vi "FPGA Main_SPI API with Waveform Library.vi"() -> ()   [LabVIEW 2014]
uses:
  <userlib>/_NI SPI IP/FPGA/Controllers/Public/Transfer Settings.ctl
  <vilib>/Platform/TimedLoop/XDataNode/timing_clust.ctl
  <vilib>/Platform/TimedLoop/XDataNode/nitl_modes.ctl
  <vilib>/Platform/TimedLoop/XDataNode/wakeup.ctl
  <vilib>/SPI API/SPIAPI/DIO/SPI Digital IO Lines.ctl
  <vilib>/SPI API/SPIAPI/DIO/SPI DIO Enable Lines.ctl
  <vilib>/rvi/Emulation/niFpgaGetClockAttributes.vi
  <vilib>/rvi/Emulation/niFpgaSctlEmulationGetInTimedLoop.vi
  <vilib>/rvi/Emulation/niFpgaEmulationReportErrorSimple.vi
  <vilib>/rvi/Emulation/niFpgaProcessEmulError.vi
  <vilib>/rvi/Emulation/niFpgaCriticalErrorInLSC.vi
  <vilib>/rvi/interface/RandomDataEmulation/niFpgaRandomDataHandleErrors.vi
  <vilib>/Platform/TimedLoop/XDataNode/XDataNode.xnode
  <vilib>/rvi/DataTransferAndStorage/Container/XNode/niFpgaContainer.xnode
  <vilib>/rvi/interface/RandomDataEmulation/nirviRandomDataFpgaReadWriteTemplate.vi
  <vilib>/Platform/TimedLoop/XDataNode/XDNodeRunTimeDep.lvlib
  <userlib>/_NI SPI IP/FPGA/Controllers/NI SPI IP FPGA.lvlib
panel:
  in  "SPI PHY Settings":T1={"Divide Value"=10, "Transfer Length (bits)"=16, "CS Asserted Polarity"=FALSE, "Clock Polarity (CPOL)"=FALSE, "Clock Phase (CPHA)"=FALSE, "Lengthen MISO Setup"=FALSE, "Direction Change Bit"=0, "MOSI Starts as Output"=FALSE, "Tristatable MOSI"=FALSE} {"Direction Change Bit" max=64 step=1; "Transfer Length (bits)" min=1 max=64 step=1}
  out "FPGA Error":errorcluster
  out "Finished":bool
  in  "stop":bool
  out "Module Underflow":bool
  out "Acq Loop Ticks":u32
  out "DMA FIFO Full":bool
  out "Chan Count":bool
  out "First Read":bool
  in  "Number of Channels":i32=4
  in  "Acquisition Type":enum16{"Finite Samples", "Continuous Samples"}(ring)
  in  "Samps per Chan [Finite]":i32=5120
  in  "Chan Scale Array":sgl[](array[numeric])=[0.0, 0.0, 0.0, 0.0, 0.0, 0.0, 0.0, 0.0, 0.0, 0.0, 0.0, 0.0, 0.0, 0.0, 0.0, 0.0, 0.0, 0.0, 0.0, 0.0, 0.0, 0.0, 0.0, 0.0, 0.0, 0.0, 0.0, 0.0, 0.0, 0.0, 0.0, 0.0, 0.0, 0.0, 0.0, 0.0, 0.0, 0.0, 0.0, 0.0]
  out "oclk mult":u32
  out "oclk div":u32
  out "oclk freq":u32
  in  "data rate (S/s)":u32
  # "Array size fixed at 40\nelements but may be \nexpanded if needed"
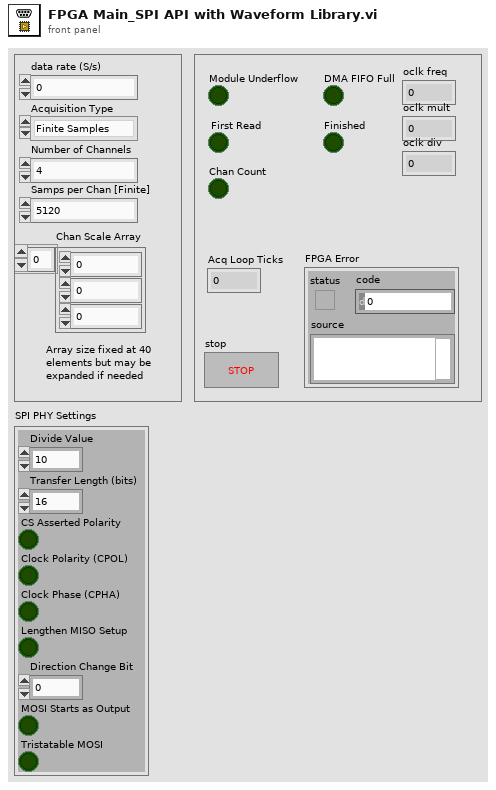
[diagram p1: front panel]
types:
  T1 = typedef "NI SPI IP FPGA.lvlib/Transfer Settings.ctl" = cluster{"Divide Value":u8, "Transfer Length (bits)":u8, "CS Asserted Polarity":bool, "Clock Polarity (CPOL)":bool, "Clock Phase (CPHA)":bool, "Lengthen MISO Setup":bool, "Direction Change Bit":u8, "MOSI Starts as Output":bool, "Tristatable MOSI":bool}
  T2 = typedef "SPI DIO Enable Lines.ctl" = cluster{"SCLK_en":refnum<k21>, "MISO_en":refnum<k21>, "MOSI_en":refnum<k21>, "CS0_en":refnum<k21>, "CS1_en":refnum<k21>, "CS2_en":refnum<k21>, "CS3_en":refnum<k21>, "CS4_en":refnum<k21>, "CS5_en":refnum<k21>}
  T3 = typedef "SPI Digital IO Lines.ctl" = cluster{"SCLK":refnum<k21>, "MISO":refnum<k21>, "MOSI":refnum<k21>, "CS 0":refnum<k21>, "CS 1":refnum<k21>, "CS 2":refnum<k21>, "CS 3":refnum<k21>, "CS 4":refnum<k21>, "CS 5":refnum<k21>}
  T4 = typedef "Internal Data (SPI API).ctl" = cluster{"DLU To SPI Engine Data FIFO":refnum<k21>, "SPI Engine to DLU Data FIFO":refnum<k21>, "Data to SPI Engine (Cache) Register":refnum<k21>, "SPI PHY Settings to SPI Engine (Cahche) Register":refnum<k21>}
  T5 = typedef "XDNodeRunTimeDep.lvlib/timing_clust.ctl" = cluster{"Expected End [f-1]":u64, "Actual End [f-1]":u64, "Finished Late? [f-1]":bool, "Expected End [i-1]":u64, "Actual End [i-1]":u64, "Finished Late? [i-1]":bool, "Expected Start [i]":u64, "Actual Start [i]":u64, "Expected Start [f]":u64, "Actual Start [f]":u64, "Source Name":string, "Structure Name":string, "Period":i64, "Deadline":i64, "Offset":i64, "Start":i64, "Priority":i32, "Timeout":i32, "Mode":T6, "Wakeup Reason":T7, "Error":errorcluster, "Source Type":string, "Secondary Source Type":string, "Global End Time":u64, "Global Start Time":u64, "Frame Duration":u64, "Iteration Duration":u64, "Assigned CPU":i32, "I/O Scan Engine Mode":u32}
  T6 = typedef "XDNodeRunTimeDep.lvlib/nitl_modes.ctl" = enum32{"No Change", "Process missed periods, maintain original phase", "Discard missed periods, maintain original phase", "Process missed periods, ignore original phase", "Discard missed periods, ignore original phase"}
  T7 = typedef "XDNodeRunTimeDep.lvlib/wakeup.ctl" = enum32{"Normal", "Aborted", "Asynchronous wakeup", "Timing source error", "Timed loop error", "Timeout"}
  T8 = typedef "SPI Response Information.ctl" = cluster{"Data to Node":u64, "Node Id":u16}
  T9 = typedef "NI SPI IP FPGA.lvlib/Spi Master Inputs.ctl" = cluster{"MISO":bool}
  T10 = typedef "NI SPI IP FPGA.lvlib/Spi Master Outputs.ctl" = cluster{"Chip Select":bool, "Clock":bool, "MOSI":bool, "MOSI OE":bool}
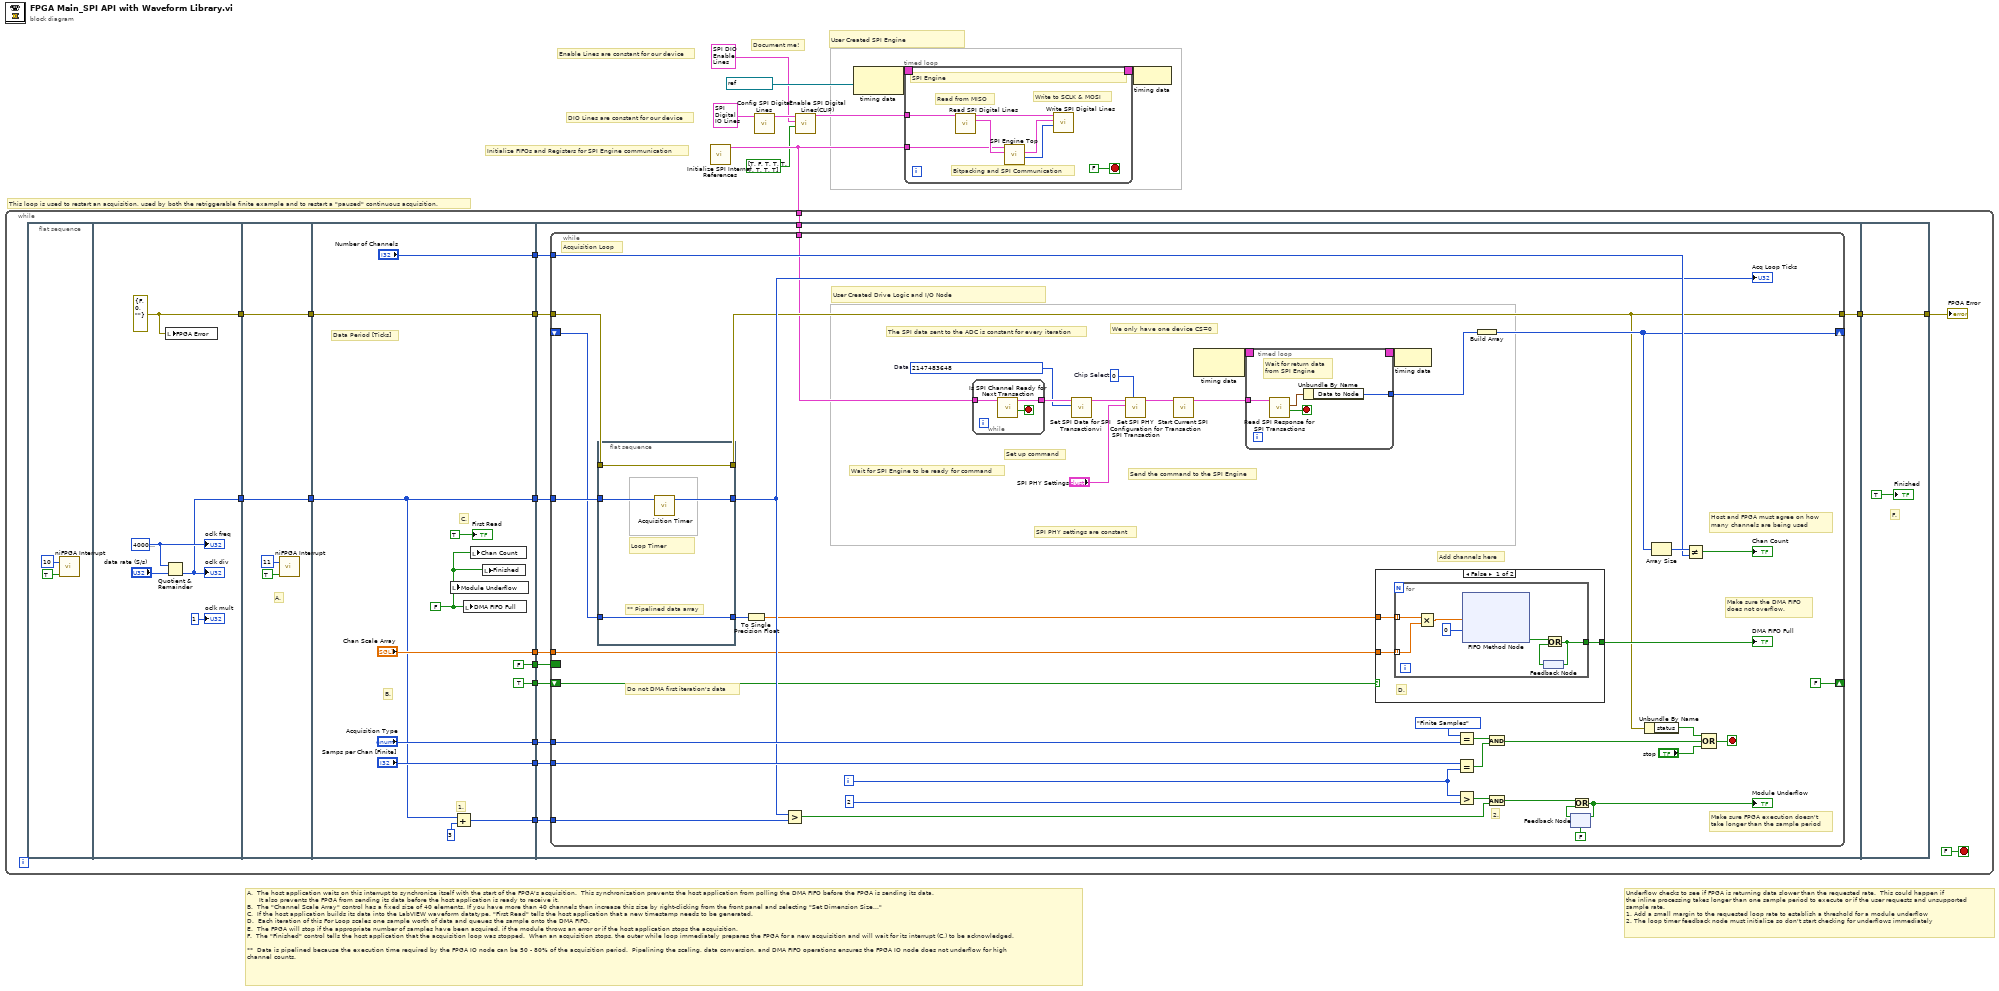
[diagram p0: block diagram]
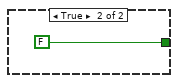
[diagram p2: hidden frame]
diagram:
  # "Initialize FIFOs and Registers for SPI Engine communication"
  # "Enable Lines are constant for our device"
  # "DIO Lines are constant for our device"
  # "Document me!"
  # "User Created SPI Engine"
  # "Underflow checks to see if FPGA is returning data slower than the requested rate.  This could happen if\nthe inline processing takes longer than one sample period to execute or if the user requests and unsupported\nsample rate.\n1. Add a small margin to the requested loop rate to establish a threshold for a module underflow \n2. The loop timer feedback node must initialize so don't start checking for underflows immediately"
  # "A.  The host application waits on this interrupt to synchronize itself with the start of the FPGA's acquisition.  This synchronization prevents the host application from polling the DMA FIFO before the FPGA is sending its data.\n      It also prevents the FPGA from sending its data before the host application is ready to receive it.\nB.  The \"Channel Scale Array\" control has a fixed size of 40 elements. If you have more than 40 channels then increase this size by right-clicking from the front panel and selecting \"Set Dimension Size...\"\nC.  If the host application builds its data into the LabVIEW waveform datatype, \"First Read\" tells the host application that a new timestamp needs to be generated.\nD.  Each iteration of this For Loop scales one sample worth of data and queues the sample onto the DMA FIFO.  \nE.  The FPGA will stop if the appropriate number of samples have been acquired, if the module throws an error or if the host application stops the acquisition.  \nF.  The \"Finished\" control tells the host application that the acquisition loop was stopped.  When an acquisition stops, the outer while loop immediately prepares the FPGA for a new acquisition and will wait for its interrupt (C.) to be acknowledged. \n\n**  Data is pipelined because the execution time required by the FPGA IO node can be 50 - 80% of the acquisition period.  Pipelining the scaling, data conversion, and DMA FIFO operations ensures the FPGA IO node does not underflow for high\nchannel counts."
  # "This loop is used to restart an acquisition, used by both the retriggerable finite example and to restart a \"paused\" continuous acquisition."
  n1 = call <vilib>:"Initialize SPI Internal References.vi"() -> ("SPI API References"=w2:T4)  [unwired: 10 in, 1 out]
  n2 = while {
    tunnel: w2 -> [w10]
    stop <- FALSE stop-if-true
    n3 = flat-sequence {
      tunnel: [w30] -> w17
      tunnel: [w29] -> w13
      tunnel: w17 -> [w35]
      tunnel: [w35] -> w16
      tunnel: [w34] -> w14
      tunnel: w13 -> [w34]
      tunnel: ["Number of Channels"] -> w26
      tunnel: ["Chan Scale Array"] -> w25
      tunnel: ["Acquisition Type"] -> w24
      tunnel: ["Samps per Chan [Finite]"] -> w23
      tunnel: [w39] -> w22
      tunnel: [w43] -> w21
      tunnel: [TRUE] -> w20
      tunnel: w16 -> [w40]
      tunnel: [w40] -> w15
      tunnel: w14 -> [w39]
      tunnel: [FALSE] -> w12
      tunnel: w26 -> [w60]
      tunnel: w25 -> [w57]
      tunnel: w24 -> [w56]
      tunnel: w23 -> [w55]
      tunnel: w22 -> [w58]
      tunnel: w21 -> [w54]
      tunnel: w20 -> [w53]
      tunnel: [w52] -> w18
      tunnel: w15 -> [w59]
      tunnel: w12 -> [w51]
      tunnel: w10 -> [w50]
      tunnel: [w131] -> w19
      tunnel: w18 -> [w131]
      frame #0 {
        n4 = call <vilib>:"niFPGA Interrupt.vi"("Wait Until Cleared (F)"=TRUE ("Wait Until Cleared"), "IRQ Number (0)"=u8 10 ("IRQ Number")) -> ()  [unwired: 1 in]
      }
      frame #1 {
        w30 = errorcluster {"status"=FALSE, "code"=0, "source"=""} ("FPGA Error")
        w31 = u32 40000000 ("oclk freq")
        n5 = Quotient & Remainder(x=w31, y="data rate (S/s)") -> (floor(x/y)=w29:u32)  [unwired: 1 out]
        "oclk div" <- w29
        n6 = local write "FPGA Error"(w30) -> ()
        "oclk mult" <- u32 1 ("oclk mult")
        "oclk freq" <- w31
      }
      frame #2 {
        # "A."
        n7 = call <vilib>:"niFPGA Interrupt.vi"("Wait Until Cleared (F)"=TRUE ("Wait Until Cleared"), "IRQ Number (0)"=u8 11 ("IRQ Number")) -> ()  [unwired: 1 in]
      }
      frame #3 {
        w48 = FALSE ("Module Underflow")
        # "Data Period [Ticks]"
        # "1."
        # "C."
        # "B."
        n8 = local write "Module Underflow"(w48) -> ()
        n9 = Add(x=w39, y=u32 3) -> (x+y=w43:u32)
        n10 = local write "DMA FIFO Full"(w48) -> ()
        n11 = local write "Chan Count"(w48) -> ()
        n12 = local write "Finished"(w48) -> ()
        "First Read" <- TRUE ("First Read")
      }
      frame #4 {
        n13 = while {
          tunnel: w56 -> [w97]
          tunnel: w55 -> [w96]
          shift-right: [w75] -> _
          shift-left: _ -> [w88]
          tunnel: w60 -> [w98]
          tunnel: w59 -> [w90]
          tunnel: [w72] -> w52
          tunnel: w58 -> [w95]
          tunnel: w54 -> [w91]
          tunnel: w57 -> [w87]
          shift-right: [FALSE] -> _
          shift-left: w53 -> [w86]
          border: w51 -> [_]
          tunnel: w50 -> [w61]
          i -> [w84]
          stop <- w102 stop-if-true
          w65 = u8 0  # Chip Select
          w67 = u64 2147483648  # Data
          # "SPI PHY settings are constant"
          # "Send the command to the SPI Engine"
          # "We only have one device CS=0"
          # "The SPI data sent to the ADC is constant for every iteration"
          # "Set up command"
          # "Wait for SPI Engine to be ready for command"
          # "User Created Drive Logic and I/O Node"
          # "Add channels here"
          # "2."
          # "Do not DMA first iteration's data"
          # "Host and FPGA must agree on how \nmany channels are being used"
          # "Acquisition Loop"
          # "Make sure the DMA FIFO\ndoes not overflow."
          # "Make sure FPGA execution doesn't\ntake longer than the sample period"
          n14 = flat-sequence {
            tunnel: w95 -> [w128]
            tunnel: [w130] -> w72
            tunnel: w90 -> [w130]
            tunnel: [w127] -> w89
            tunnel: [w129] -> w74
            tunnel: w88 -> [w129]
            frame #0 {
              # "Loop Timer"
              # "** Pipelined data array"
              n15 = call <vilib>:"Acquisition Timer.vi"("Loop Time (Ticks)"=w128) -> ("Actual Time (Ticks)"=w127:u32)  [unwired: 10 in]
            }
          }
          n16 = To Single Precision Float(number=w74) -> (single precision float=w73:sgl[])
          n17 = Greater?(x=w89, y=w91) -> (0:w94:bool)
          n18 = while {
            tunnel: w61 -> [w114]
            tunnel: [w113] -> w68
            stop <- w115 stop-if-true
            n19 = call <vilib>:"Is SPI Channel Ready for Next Transaction.vi"("Private Data In"=w114) -> ("SPI Channel Ready"=w115:bool, "Private Data Out"=w113:T4)  [unwired: 7 in, 2 out]
          }
          n20 = call <vilib>:"Set SPI Data for SPI Transactionvi.vi"("Data In"=w67, "Private Data In"=w68) -> ("Private Data Out"=w66:T4)  [unwired: 8 in, 1 out]
          n21 = call <vilib>:"Set SPI PHY Configuration for SPI Transaction.vi"("Chip Select"=w65, "SPI PHY Settings"="SPI PHY Settings", "Private Data In"=w66) -> ("Private Data Out"=w64:T4)  [unwired: 7 in, 1 out]
          n22 = call <vilib>:"Start Current SPI Transaction.vi"("Private Data In"=w64) -> ("Private Data Out"=w63:T4)  [unwired: 8 in, 2 out]
          n23 = node-c288() -> (w71:T5)  [unwired: 1 in]
          n24 = timed-loop {
            timing: w71 -> [_]
            timing-out: [_] -> w70
            tunnel: w63 -> [w108]
            tunnel: [w105] -> w62
            stop <- w107 stop-if-true
            # "Wait for return data\nfrom SPI Engine"
            n25 = call <vilib>:"Read SPI Response for SPI Transactions.vi"("Private Data In"=w108) -> ("Read Data Valid?"=w107:bool, "Read Data"=w106:T8)  [unwired: 7 in, 2 out]
            n26 = Unbundle By Name(w106) -> ("Data to Node"=w105:u64)
          }
          n27 = case shown="False" w86 {
            tunnel: [w118 FALSE] -> w101
            tunnel: w73 -> [w117 _]
            tunnel: w87 -> [w116 _]
            frame False {
              # "D."
              n28 = for {
                tunnel: [w124] -> w118
                tunnel: w117 -> [w123] mode=indexing
                tunnel: w116 -> [w119] mode=indexing
                n29 = Multiply(x=w123, y=w119) -> (x*y=w120:sgl)
                n30 = xnode ("FIFO Method Node")("Element"=w120, "Timeout"=0) -> ("Timed Out?"=w121:bool)  [unwired: 1 in, 1 out]
                n31 = feedback #1() -> (w125:bool)
                n32 = Or(x=w121, y=w125) -> (x .or. y?=w124:bool)
                n33 = feedback-in #1(w124) -> ()
              }
            }
            frame True {
            }
          }
          "DMA FIFO Full" <- w101
          n34 = node-c288(w70) -> ()
          n35 = Equal?(x=enum16{"Finite Samples", "Continuous Samples"}."Finite Samples" ("y"), y=w97) -> (x = y?=w78:bool)
          n36 = Equal?(x=w96, y=w84) -> (x = y?=w77:bool)
          n37 = Greater?(x=w84, y=2) -> (0:w93:bool)
          n38 = Build Array(w62) -> (w75:u64[])
          n39 = And(x=w78, y=w77) -> (x .and. y?=w76:bool)
          n40 = And(x=w93, y=w94) -> (x .and. y?=w80:bool)
          n41 = feedback #2(FALSE) -> (w82:bool)
          n42 = Or(x=w80, y=w82) -> (x .or. y?=w79:bool)
          "Module Underflow" <- w79
          n43 = feedback-in #2(w79) -> ()
          n44 = Unbundle By Name(w72) -> ("status"=w83:bool)
          n45 = Array Size(array=w75) -> (size(s)=w100:i32)
          n46 = Not Equal?(x=w100, y=w98) -> (x != y?=→"Chan Count":bool)
          n47 = Compound Arithmetic op=OR(w83, w76, "stop") -> (w102:bool)
          "Acq Loop Ticks" <- w89
        }
      }
      frame #5 {
        # "F."
        "Finished" <- TRUE ("Finished")
      }
    }
    "FPGA Error" <- w19
  }
  n48 = call <vilib>:"Config SPI Digital Lines.vi"("SPI DIO Lines"=T3 {"SCLK"="sbRIO-9651 Socket\\PMOD1_Pin4_out", "MISO"="sbRIO-9651 Socket\\PMOD1_Pin3_in", "MOSI"="sbRIO-9651 Socket\\PMOD1_Pin2_out", "CS 0"="sbRIO-9651 Socket\\PMOD1_Pin1_out", "CS 1"="sbRIO-9651 Socket\\PMOD1_Pin1_out", "CS 2"="sbRIO-9651 Socket\\PMOD1_Pin1_out", "CS 3"="sbRIO-9651 Socket\\PMOD1_Pin1_out", "CS 4"="sbRIO-9651 Socket\\PMOD1_Pin1_out", "CS 5"="sbRIO-9651 Socket\\PMOD1_Pin1_out"}) -> ("Chip Select DIO Lines"=w5:T3)  [unwired: 9 in, 1 out]
  n49 = call <vilib>:"Enable SPI Digital Lines(CLIP).vi"("Enable"=bool[] [TRUE, FALSE, TRUE, TRUE, TRUE, TRUE, TRUE, TRUE, TRUE], "Enable Lines"=T2 {"SCLK_en"="sbRIO-9651 Socket\\PMOD1_Pin4_enable", "MISO_en"="sbRIO-9651 Socket\\PMOD1_Pin3_enable", "MOSI_en"="sbRIO-9651 Socket\\PMOD1_Pin2_enable", "CS0_en"="sbRIO-9651 Socket\\PMOD1_Pin1_enable", "CS1_en"="sbRIO-9651 Socket\\PMOD1_Pin1_enable", "CS2_en"="sbRIO-9651 Socket\\PMOD1_Pin1_enable", "CS3_en"="sbRIO-9651 Socket\\PMOD1_Pin1_enable", "CS4_en"="sbRIO-9651 Socket\\PMOD1_Pin1_enable", "CS5_en"="sbRIO-9651 Socket\\PMOD1_Pin1_enable"}, "SPI DIO Lines"=w5) -> ("Chip Select DIO Lines"=w7:T3)  [unwired: 7 in, 1 out]
  n50 = node-c288(refnum<k21> "120MHz" ("Source Name")) -> (w9:T5)
  n51 = timed-loop {
    timing: w9 -> [_]
    timing-out: [_] -> w8
    tunnel: w7 -> [w135]
    tunnel: w2 -> [w133]
    stop <- FALSE stop-if-true
    # "Bitpacking and SPI Communication"
    # "Write to SCLK & MOSI"
    # "Read from MISO"
    # "SPI Engine"
    n52 = call <vilib>:"Read SPI Digital Lines.vi"("Chip Select DIO Lines"=w135) -> ("Chip Select DIO Lines Out"=w139:T3, "SPI Read Data"=w138:T9)  [unwired: 12 in, 1 out]
    n53 = call <vilib>:"SPI Engine Top.vi"("SPI Read Data"=w138, "SPI API References"=w133) -> ("Chip Select ID"=w136:u8, "SPI DIO Output"=w137:T10)  [unwired: 6 in, 2 out]
    n54 = call <vilib>:"Write SPI Digital Lines.vi"("CS Index"=w136, "spi output"=w137, "Chip Select DIO Lines"=w139) -> ()  [unwired: 7 in, 2 out]
  }
  n55 = node-c288(w8) -> ()
